vi "Initialize Instrument.vi"(8 "error in (no error)":errorcluster, 10 "Reset":bool, 11 "MXA in":refnum<class "MXA.lvclass">) -> (0 "error out":errorcluster, 3 "MXA out":refnum<class "MXA.lvclass">)   [LabVIEW 2020, in "MXA.lvclass"]
uses:
  MXA.lvclass
  C:/Sandbox/RF Bench/Source Code/WiSpry Test Framework/Instruments/Instrument.lvclass
  C:/Sandbox/RF Bench/Source Code/WiSpry Test Framework/Instruments/Spectrum Analyzer/Spectrum Analyzer.lvclass
  Instrument.lvclass/Instrument.ctl
  Spectrum Analyzer.lvclass/Spectrum Analyzer.ctl
  <vilib>/Utility/config.llb/Read Key (Double).vi
  Instrument.lvclass
  <instrlib>/Agilent MXA Series/Agilent MXA Series.lvlib
  Spectrum Analyzer.lvclass
  <vilib>/Utility/config.llb/NI_LVConfig.lvlib
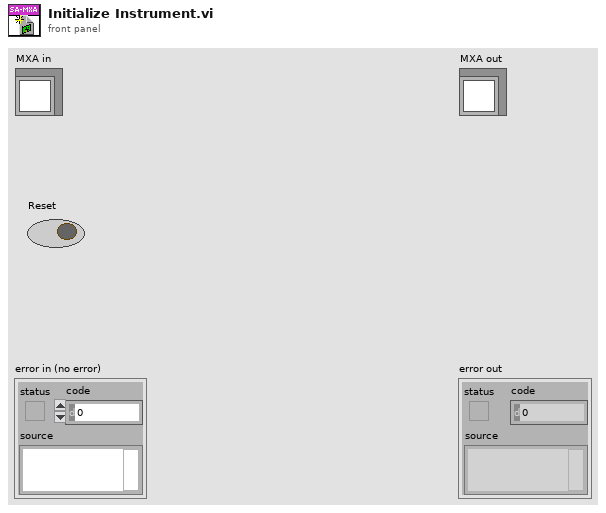
[diagram p1: front panel]
types:
  T1 = typedef "NI_LVConfig.lvlib/Config Data RefNum.ctl" = refnum<k1>
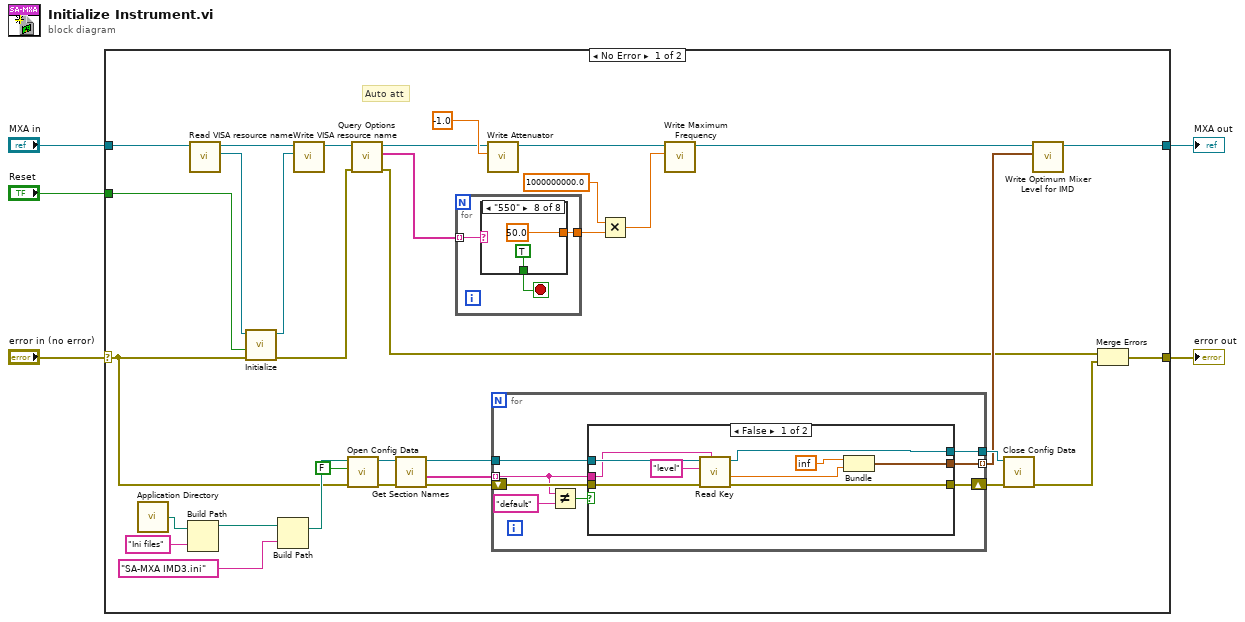
[diagram p0: block diagram]
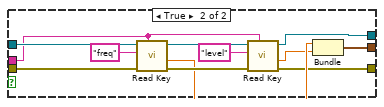
[diagram p2: hidden frame]
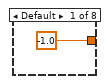
[diagram p3: hidden frame]
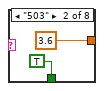
[diagram p4: hidden frame]
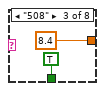
[diagram p5: hidden frame]
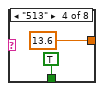
[diagram p6: hidden frame]
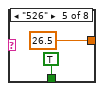
[diagram p7: hidden frame]
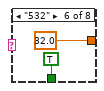
[diagram p8: hidden frame]
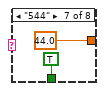
[diagram p9: hidden frame]
diagram:
  n1 = case shown="No Error" "error in (no error)" {
    selector: "error in (no error)" -> [w12 w88]
    tunnel: "MXA in" -> [w35 w87]
    tunnel: [w6 w88] -> w4
    tunnel: [w11 w87] -> w3
    tunnel: "Reset" -> [w39 _]
    frame No Error {
      # "Auto att"
      n2 = call <vilib>:"Application Directory.vi"() -> ("Application Directory"=w25:path)
      n3 = Build Path(base path=w25, name or relative path="Ini files") -> (appended path=w24:path)
      n4 = call "Read VISA resource name.vi"("Instrument in"=w35) -> ("VISA resource name"=w38:refnum<visa-resource-name>, "Instrument out"=w32:refnum<class "MXA.lvclass">)  [unwired: 9 in]
      n5 = call <instrlib>:"Initialize.vi"("error in (no error)"=w12, "Reset (True)"=w39, "VISA resource name"=w38) -> ("error out"=w30:errorcluster, "VISA resource name out"=w34:refnum<visa-resource-name>)  [unwired: 7 in]
      n6 = Build Path(base path=w24, name or relative path="SA-MXA IMD3.ini") -> (appended path=w15:path)
      n7 = call "Write VISA resource name.vi"("VISA resource name"=w34, "Instrument in"=w32) -> ("Instrument out"=w33:refnum<class "MXA.lvclass">)  [unwired: 9 in]
      n8 = call <vilib>:"Open Config Data.vi"("error in (no error)"=w12, "create file if necessary (T)"=FALSE, "configuration file path"=w15) -> ("error out"=w22:errorcluster, "refnum"=w21:T1)  [unwired: 6 in, 1 out]
      n9 = call-dynamic "Query Options.vi"("error in (no error)"=w30, "Instrument in"=w33) -> ("error out"=w7:errorcluster, "Options"=w29:string[], "Instrument out"=w31:refnum<class "MXA.lvclass">)  [unwired: 7 in]
      n10 = call <vilib>:"Get Section Names.vi"("error in (no error)"=w22, "refnum"=w21) -> ("error out"=w20:errorcluster, "section names"=w19:string[], "refnum out"=w18:T1)  [unwired: 7 in]
      n11 = for {
        tunnel: w29 -> [w71] mode=indexing
        tunnel: [w70] -> w28
        stop <- w69 stop-if-true
        n12 = case shown="\"550\"" w71 {
          tunnel: [-1.0 ("Attenuator") 3.6 ("Attenuator") 8.4 ("Attenuator") 13.6 ("Attenuator") 26.5 ("Attenuator") 32.0 ("Attenuator") 44.0 ("Attenuator") 50.0 ("Attenuator")] -> w70
          tunnel: [_ TRUE TRUE TRUE TRUE TRUE TRUE TRUE] -> w69
          frame Default {
          }
          frame "503" {
          }
          frame "508" {
          }
          frame "513" {
          }
          frame "526" {
          }
          frame "532" {
          }
          frame "544" {
          }
          frame "550" {
          }
        }
      }
      n13 = call "Write Attenuator.vi"("Attenuator"=-1.0, "Spectrum Analyzer in"=w31) -> ("Spectrum Analyzer out"=w36:refnum<class "MXA.lvclass">)  [unwired: 9 in]
      n14 = for {
        tunnel: w19 -> [w43] mode=indexing
        tunnel: w18 -> [w44]
        shift-right: [w41] -> w17
        shift-left: w20 -> [w45]
        tunnel: [w42] -> w9 mode=indexing
        tunnel: [w40] -> w13
        n15 = Not Equal?(x=w43, y="default") -> (x != y?=w46:bool)
        n16 = case shown="False" w46 {
          tunnel: w45 -> [w56 w68]
          tunnel: w44 -> [w55 w67]
          tunnel: w43 -> [w54 w65]
          tunnel: [w48 w59] -> w42
          tunnel: [w50 w58] -> w41
          tunnel: [w49 w57] -> w40
          frame False {
            n17 = call-poly <vilib>:"Read Key.vi"("section"=w54, "error in (no error)"=w56, "key"="level", "refnum"=w55) -> ("error out"=w50:errorcluster, "value"=w51:dbl, "refnum out"=w49:T1)  [unwired: 4 in, 1 out]
            n18 = Bundle(inf, "value"=w51) -> (w48:cluster{dbl, "value":dbl})  [unwired: 1 in]
          }
          frame True {
            n19 = call-poly <vilib>:"Read Key.vi"("section"=w65, "error in (no error)"=w68, "key"="freq", "refnum"=w67) -> ("error out"=w66:errorcluster, "value"=w61:dbl, "refnum out"=w63:T1)  [unwired: 4 in, 1 out]
            n20 = call-poly <vilib>:"Read Key.vi"("section"=w65, "error in (no error)"=w66, "key"="level", "refnum"=w63) -> ("error out"=w58:errorcluster, "value"=w60:dbl, "refnum out"=w57:T1)  [unwired: 4 in, 1 out]
            n21 = Bundle("value"=w61, "value"=w60) -> (w59:cluster{"value":dbl, "value":dbl})  [unwired: 1 in]
          }
        }
      }
      n22 = Multiply(x=1000000000.0 ("y"), y=w28) -> (x*y=w26:dbl)
      n23 = call "Write Maximum Frequency.vi"("Maximum Frequency"=w26, "Spectrum Analyzer in"=w36) -> ("Spectrum Analyzer out"=w10:refnum<class "MXA.lvclass">)  [unwired: 9 in]
      n24 = call <vilib>:"Close Config Data.vi"("error in (no error)"=w17, "refnum"=w13) -> ("error out"=w8:errorcluster)  [unwired: 8 in, 1 out]
      n25 = call "Write Optimum Mixer Level for IMD.vi"("Optimum Mixer Level for IMD"=w9, "Spectrum Analyzer in"=w10) -> ("Spectrum Analyzer out"=w11:refnum<class "MXA.lvclass">)  [unwired: 9 in]
      n26 = Merge Errors(w7, w8) -> (w6:errorcluster)
    }
    frame Error {
    }
  }
  "error out" <- w4
  "MXA out" <- w3
